vi "GetNormCurrent.vi"(8 "error in (no error)":errorcluster, 9 "Norm. to temperature (°C)":dbl, 10 "Measured temperature (°C)":dbl, 11 "Measured Current":dbl format="%#_13g") -> (0 "error out":errorcluster, 2 "Normalized current":dbl)   [LabVIEW 2018]
doc: "Calculates current normilized to a user-defined temperature out of measured current and temperature.\nInsert temperature in °C, obtained current units will be equal to the units of the input current."
uses:
  <vilib>/express/express arith-compare/Formula/XNode/ExpressFormulaBlockNode.xnode
panel:
  out "Temperature [°C]":dbl
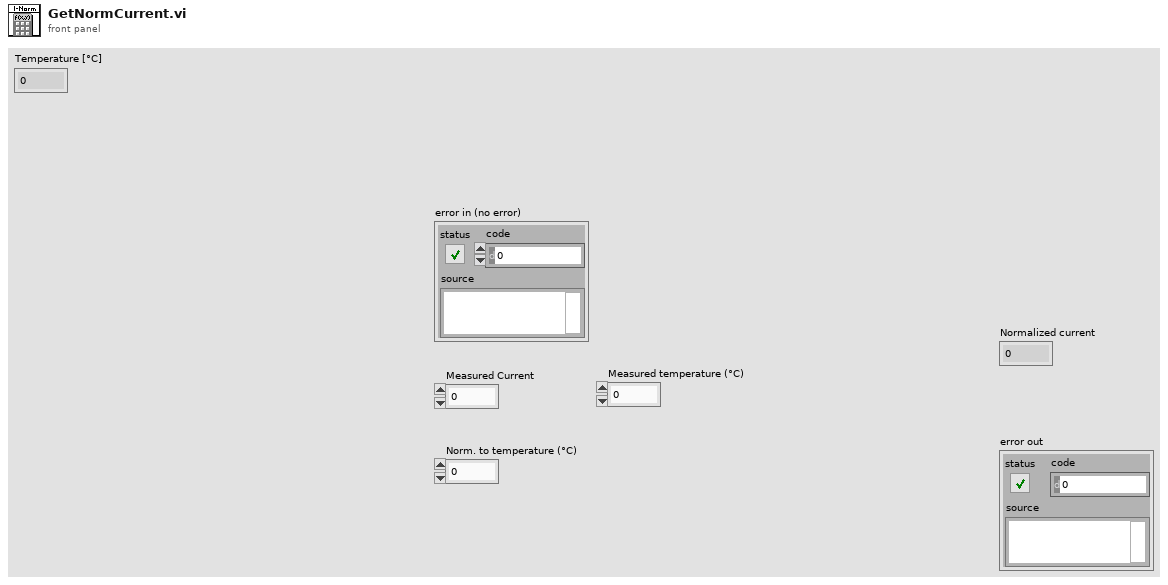
[diagram p1: front panel]
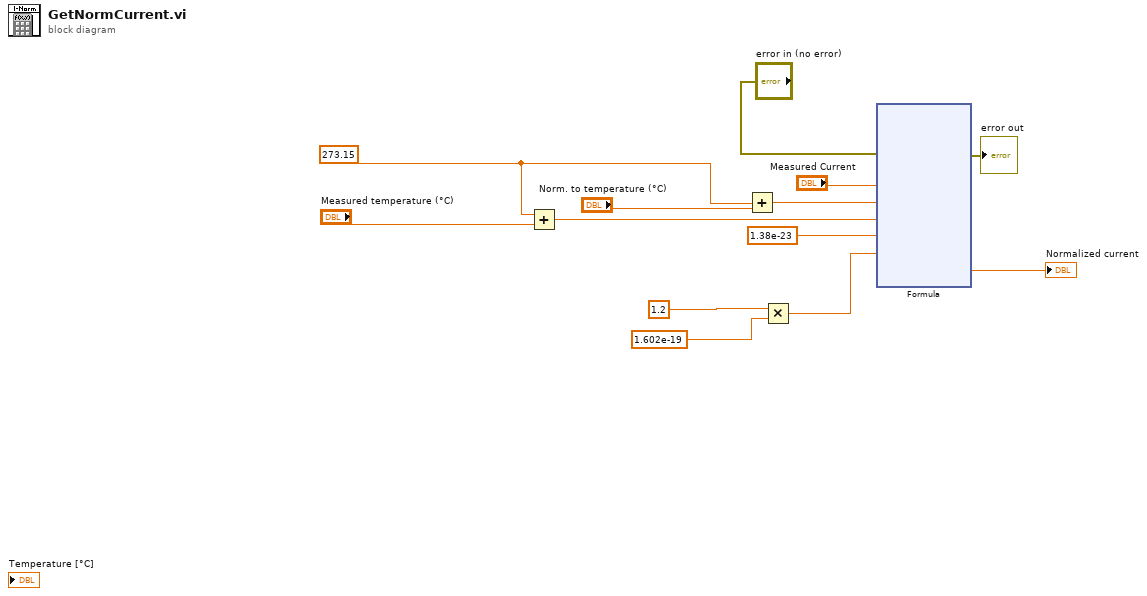
[diagram p0: block diagram]
diagram:
  w6 = 273.15
  n1 = Add(x="Measured temperature (°C)", y=w6) -> (x+y=w9:dbl)
  n2 = Add(x="Norm. to temperature (°C)", y=w6) -> (x+y=w10:dbl)
  n3 = Multiply(x=1.2, y=1.602e-19) -> (x*y=w12:dbl)
  n4 = xnode "Formula"("Current"="Measured Current", "Norm.temp"=w10, "Temperature"=w9, "k_B"=1.38e-23, "E_eff"=w12, "error in (no error)"="error in (no error)") -> ("Result"=→"Normalized current":dbl, "error out"=→"error out":errorcluster)
